vi "IsSearchGoalNode.vi"(8 "error in (no error)":errorcluster, 10 "PossibleGoalNode in":refnum<data-value>, 11 "OccupancyMap in":refnum<class "OccupancyMap.lvclass">) -> (0 "error out":errorcluster, 1 "IsGoal":bool, 2 "PossibleGoalNode out":refnum<data-value>, 3 "OccupancyMap out":refnum<class "OccupancyMap.lvclass">)   [LabVIEW 2014, in "OccupancyMap.lvclass"]
uses:
  <userlib>/AdvancedDataStructures/ClassBased/Applications/Occupancy/OccupancyMap/OccupancyMap.lvclass
  <userlib>/AdvancedDataStructures/ClassBased/GraphNode/GraphNode.lvclass
  <userlib>/AdvancedDataStructures/ClassBased/Applications/Occupancy/Cell/Cell.lvclass
  <userlib>/AdvancedDataStructures/ClassBased/Applications/Occupancy/OccupancyMap/OccupancyMap.lvclass/OccupancyMap.ctl
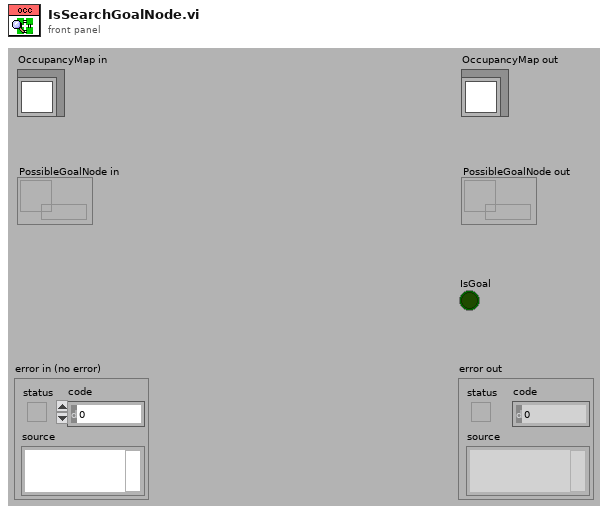
[diagram p1: front panel]
types:
  T1 = cluster{"Left":dbl, "Right":dbl, "Top":dbl, "Bottom":dbl}
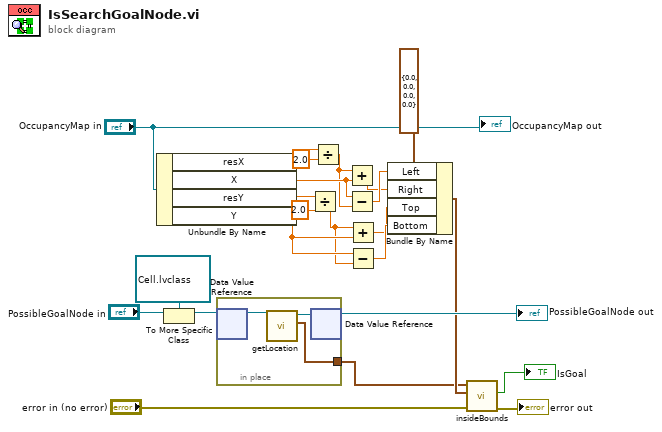
[diagram p0: block diagram]
diagram:
  n1 = Unbundle By Name("OccupancyMap in") -> ("resX"=w6:dbl, "X"=w15:dbl, "resY"=w3:dbl, "Y"=w11:dbl)
  n2 = To More Specific Class(target class=refnum<data-value> refnum ("data value reference"), reference="PossibleGoalNode in") -> (specific class reference=w20:refnum<data-value>)  [unwired: 1 in, 1 out]
  n3 = in-place {
    in-place-border: [w24] -> w7
    n4 = in-place-dvr #1(w20) -> (w26:refnum<class "Cell.lvclass">)  [unwired: 1 out]
    n5 = call <userlib>:"getLocation.vi"("Cell in"=w26) -> ("Location"=w24:cluster{"X":dbl, "Y":dbl}, "Cell out"=w25:refnum<class "Cell.lvclass">)  [unwired: 8 in, 1 out]
    n6 = in-place-dvr #1(w25) -> (→"PossibleGoalNode out":refnum<data-value>)  [unwired: 1 out]
  }
  n7 = Divide(x=w3, y=2.0) -> (x/y=w1:dbl)
  n8 = Divide(x=w6, y=2.0) -> (x/y=w4:dbl)
  n9 = Add(x=w4, y=w15) -> (x+y=w8:dbl)
  n10 = Subtract(x=w15, y=w4) -> (x-y=w9:dbl)
  n11 = Add(x=w1, y=w11) -> (x+y=w10:dbl)
  n12 = Subtract(x=w11, y=w1) -> (x-y=w12:dbl)
  n13 = Bundle By Name(cluster=T1 {"Left"=0.0, "Right"=0.0, "Top"=0.0, "Bottom"=0.0} ("Rectangle"), "Left"=w9, "Right"=w8, "Top"=w10, "Bottom"=w12) -> (w13:T1)
  n14 = call <userlib>:"insideBounds.vi"("error in (no error)"="error in (no error)", "Rectangle"=w13, "point"=w7) -> ("error out"=→"error out":errorcluster, "inside"=→"IsGoal":bool)  [unwired: 7 in]
  "OccupancyMap out" <- "OccupancyMap in"
